vi "Do Action.vi"(8 "error in (no error)":errorcluster, 9 "Display Queue":refnum<queue>, 10 "tlc_User Event Reference.ctl":T1, 11 "Initialize Application in":refnum<class "Initialize Application.lvclass">) -> (0 "error out":errorcluster)   [LabVIEW 2010, in "Initialize Application.lvclass"]
doc: "This instance of Do Action.vi is used to perform the functionality that was previously contained in the Initialize case of the consumer loop.\n\nThis function calls tlc_Initialize which will initialize all of the functional global variables that have been defined for this applicaiton, including the display module."
uses:
  Initialize Application.lvclass
  Controls/tlc_User Interface Command.ctl
  Controls/tlc_User Interface Data Type.ctl
  Controls/tlc_User Event Reference.ctl
  Initialize Application.lvclass/Initialize Application.ctl
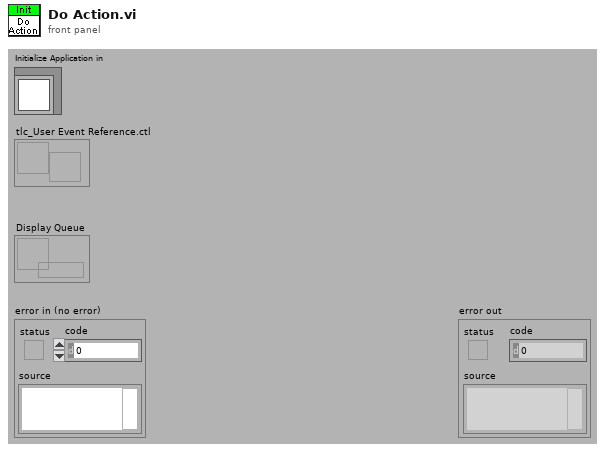
[diagram p1: front panel]
types:
  T1 = typedef "tlc_User Event Reference.ctl" = refnum<user-event>
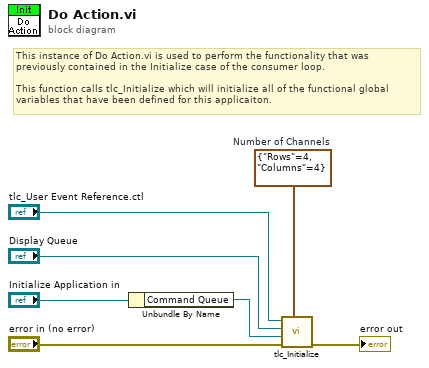
[diagram p0: block diagram]
diagram:
  w7 = cluster{"Rows":i32, "Columns":i32} {"Rows"=4, "Columns"=4}  # Number of Channels
  # "This instance of Do Action.vi is used to perform the functionality that was previously contained in the Initialize case of the consumer loop.\n\nThis function calls tlc_Initialize which will initialize all of the functional global variables that have been defined for this applicaiton."
  n1 = Unbundle By Name "Unbundle By Name"("Initialize Application in") -> ("Command Queue"=w3:refnum<queue>)
  n2 = call "tlc_Initialize.vi"("Number of Channels"=w7, "error in (no error)"="error in (no error)", "tlc_Consumer Queue Reference.ctl"=w3, "tlc_Display Queue Reference.ctl"="Display Queue", "tlc_User Event Reference.ctl"="tlc_User Event Reference.ctl") -> ("error out"=→"error out":errorcluster)  [unwired: 6 in]
